vi "SS Read Data Q.vi"(8 "error in (no error)":errorcluster, 11 "Subsystem Class in":refnum<class "Subsystem Class.lvclass">) -> (0 "error out":errorcluster, 2 "Data Q":refnum<queue>, 3 "Subsystem Class out":refnum<class "Subsystem Class.lvclass">)   [LabVIEW 2021, in "Subsystem Class.lvclass"]
uses:
  Subsystem Class.lvclass
  SS cluster Data Queue type.ctl
  Subsystem Class.lvclass/Subsystem Class.ctl
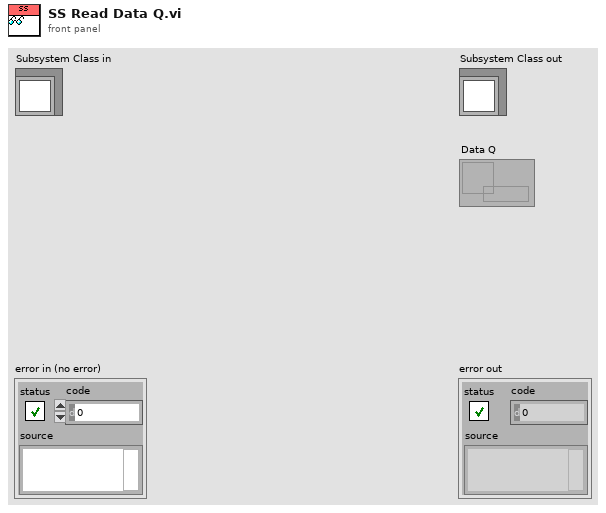
[diagram p1: front panel]
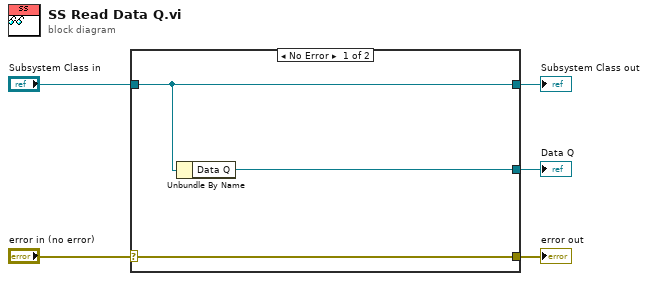
[diagram p0: block diagram]
diagram:
  n1 = case shown="No Error" "error in (no error)" {
    selector: "error in (no error)" -> [w8 w9]
    tunnel: [w8 w9] -> w4
    tunnel: [w7 w10] -> w2
    tunnel: "Subsystem Class in" -> [w7 w10]
    tunnel: [w6 _] -> w1
    frame No Error {
      n2 = Unbundle By Name(w7) -> ("Data Q"=w6:refnum<queue>)
    }
    frame Error {
    }
  }
  "error out" <- w4
  "Subsystem Class out" <- w2
  "Data Q" <- w1
